vi "GetGraphType.vi"(5 "error in (no error)":errorcluster) -> (19 "error out":errorcluster)   [LabVIEW 2020, in "Graph.lvclass"]
uses:
  <resource>/Framework/Providers/Open_GDS/UML/Graph_class/Graph.lvclass
panel:
  in  "DiagramTypeName":string
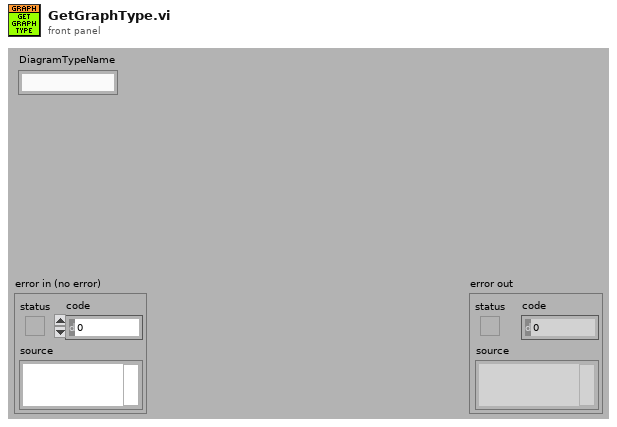
[diagram p1: front panel]
types:
  T1 = typedef "Graph.lvclass/ClassAttributes.ctl" = cluster{"NODE_PROT":refnum<class "AbstractNode.lvclass">[], "NodeNames":string[], "EDGE_PROT":refnum<class "AbstractEdge.lvclass">[], "EdgeNames":string[], "GraphTypes":refnum<class "Graph.lvclass">[], "GraphTypeNames":string[], "NodeTypes":refnum<class "AbstractNode.lvclass">[], "EdgeTypes":refnum<class "AbstractEdge.lvclass">[], "NodeTypeNames":string[], "EdgeTypeNames":string[]}
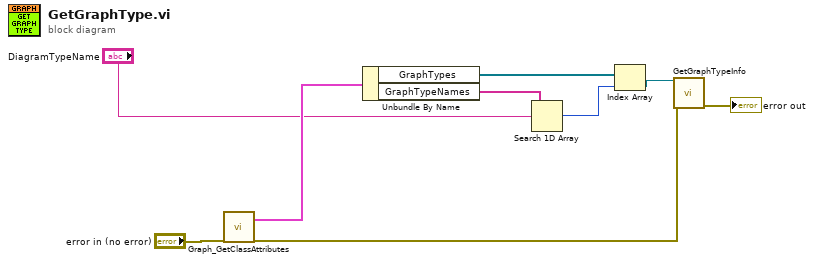
[diagram p0: block diagram]
diagram:
  n1 = call <resource>:"Graph_GetClassAttributes.vi"("error in (no error)"="error in (no error)") -> ("Class attribute"=w8:T1, "error out"=w2:errorcluster)  [unwired: 15 in, 2 out]
  n2 = Unbundle By Name(w8) -> ("GraphTypes"=w5:refnum<class "Graph.lvclass">[], "GraphTypeNames"=w7:string[])
  n3 = Search 1D Array(1D array=w7, element="DiagramTypeName") -> (index of element=w4:i32)  [unwired: 1 in]
  n4 = Index Array(array=w5, index=w4) -> (element=w3:refnum<class "Graph.lvclass">)
  n5 = call-dynamic "GetGraphTypeInfo.vi"("reference in"=w3, "error in (no error)"=w2) -> ("error out"=→"error out":errorcluster)  [unwired: 12 in, 5 out]
